vi "Post Status Update.vi"(6 "Authorization":T1[](array[typedef]), 7 "Color":enum16{"Green", "Yellow", "Red"}(ring), 8 "error in (no error)":errorcluster, 9 "Text":string, 10 "Title":string, 11 "Project":string) -> (0 "error out":errorcluster, 2 "gid":string)   [LabVIEW 2016]
uses:
  <vilib>/addons/_JKI.lib/REST Client/classes/REST Client/HTTP Header.ctl
  <vilib>/addons/_JKI.lib/REST Client/classes/REST Client/REST Client.lvclass
  <vilib>/addons/_JKI.lib/Serialization/JSON/JKI JSON Serialization.lvlib
panel:
  out "Response body":string
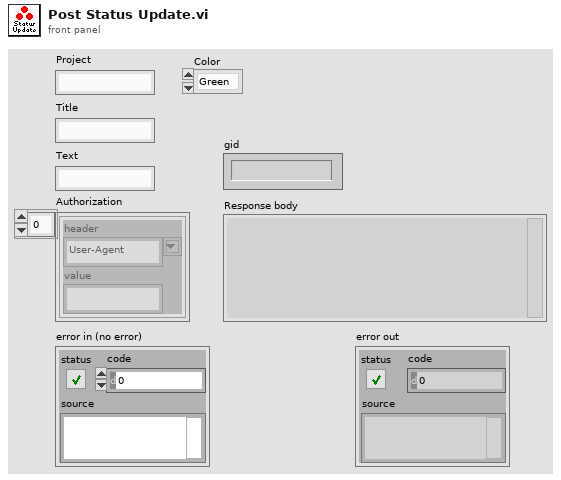
[diagram p1: front panel]
types:
  T1 = typedef "REST Client.lvlib/REST Client.lvclass/HTTP Header.ctl" = cluster{"header":string, "value":string}
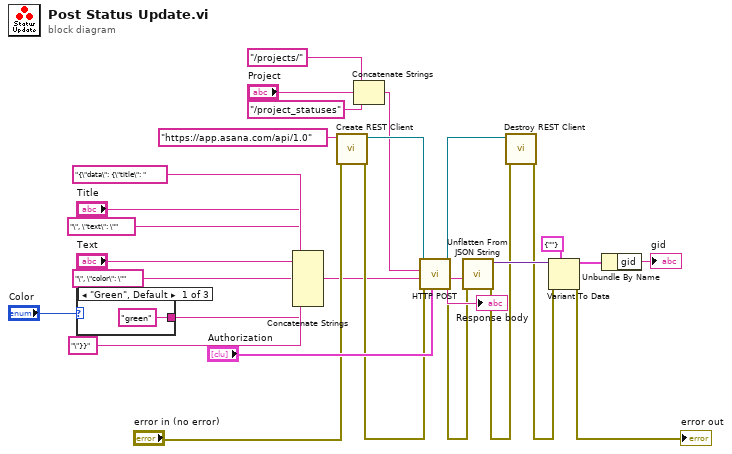
[diagram p0: block diagram]
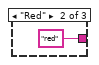
[diagram p2: hidden frame]
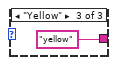
[diagram p3: hidden frame]
diagram:
  n1 = case shown="\"Green\", Default" "Color" {
    tunnel: ["green" "red" "yellow"] -> w1
    frame "Green", Default {
    }
    frame "Red" {
    }
    frame "Yellow" {
    }
  }
  n2 = Concatenate Strings("{\"data\": {\"title\": ", "Title", "\", \"text\": \"" ("string"), "Text", "\", \"color\": \"", w1, "\"}}" ("string")) -> (w22:string)
  n3 = call <vilib>:"Create REST Client.vi"("error in (no error)"="error in (no error)", "Base URL"="https://app.asana.com/api/1.0") -> ("error out"=w23:errorcluster, "REST Client out"=w26:refnum<class "REST Client.lvclass">)  [unwired: 8 in]
  n4 = Concatenate Strings("/projects/" ("Path"), "Project", "/project_statuses") -> (w8:string)
  n5 = call-dynamic "HTTP POST.vi"("request specific headers"="Authorization", "error in (no error)"=w23, "Request body"=w22, "Path"=w8, "REST Client in"=w26) -> ("error out"=w19:errorcluster, "Response body"=w20:string, "REST Client out"=w25:refnum<class "REST Client.lvclass">)  [unwired: 1 in, 3 out]
  "Response body" <- w20
  n6 = call <vilib>:"Unflatten From JSON String.vi"("error in (no error)"=w19, "JSON String"=w20) -> ("error out"=w18:errorcluster, "Variant"=w21:variant)  [unwired: 8 in]
  n7 = call-dynamic "Destroy REST Client.vi"("error in (no error)"=w18, "REST Client in"=w25) -> ("error out"=w17:errorcluster)  [unwired: 9 in]
  n8 = Variant To Data(error in=w17, type=cluster{"gid":string} {"gid"=""}, Variant=w21) -> (data=w14:cluster{"gid":string}, error out=→"error out":errorcluster)
  n9 = Unbundle By Name(w14) -> ("gid"=→"gid":string)
